vi "fgv_DSP_visa.vi"(7 "action":T1=enum."on", 8 "error in":errorcluster) -> (0 "error out":errorcluster)   [LabVIEW 2019]
uses:
  _ctrl/DSP_action.ctl
  _ctrl/rw.ctl
  _ctrl/init-r-stop.ctl
  SubVIs/common/cmd_err.ctl
  SubVIs/common/Glob_Ref.vi
panel:
  out "Waveform Chart":dbl(graph)
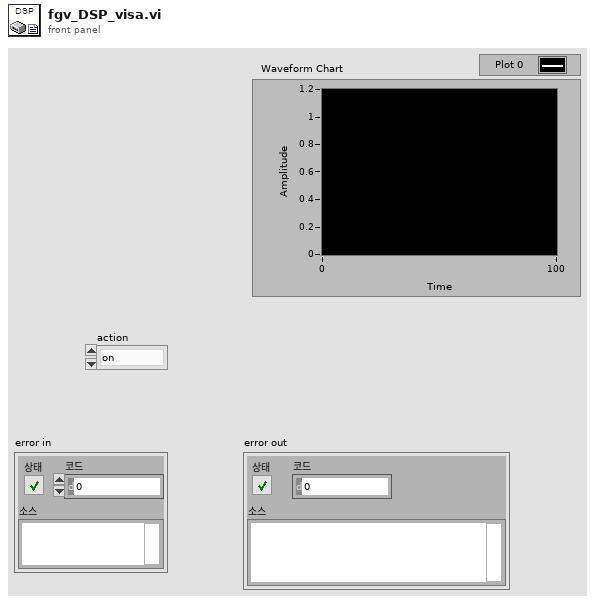
[diagram p1: front panel]
types:
  T1 = typedef "DSP_action.ctl" = enum16{"False", "cont", "on", "off", "discont", "protection", "protection_seq", "preread", "level_seq", "level_m", "read", "stop", "exit"}
  T2 = typedef "rw.ctl" = enum16{"read", "write"}
  T3 = enum16{"DL950", "BP4610", "DSP1500", "cDAQ-AI", "cDAQ-AO", "cDAQ-DO"}
  T4 = typedef "init-r-stop.ctl" = enum16{"ini", "read", "stop"}
  T5 = typedef "cmd_err.ctl" = enum16{"close", "open", "default"}
  T6 = typedef "DSP_config.ctl" = cluster{"Port":refnum<visa-resource-name>, "OVP Level":dbl, "OCP Level":dbl, "Current":dbl, "Voltage":dbl}
  T7 = typedef "DSP_retrun.ctl" = cluster{"voltage":dbl, "current":dbl, "Read Data":string}
  T8 = typedef "cap_config.ctl" = cluster{"Test Mode":enum32{"6.3.2 저온 작동/방치 시험", "6.3.3 고온 작동/방치 시험", "6.3.4 온도 싸이클 시험", "6.3.6 온습도 싸이클 시험", "6.3.8 결로 시험", "6.3.9 빙결 시험", "ON/OFF 동작시험"}, "ON time[ms]":dbl, "OFF time[ms]":dbl, "1. 작동시간[분]":dbl, "2. 미작동시간[분]":dbl, "3. 작동시간[분]":dbl, "level[V]":dbl, "duty":dbl, "Freq":dbl, "Voltage+[V]":dbl, "Voltage-[V]":dbl, "Current+[A]":dbl, "Current-[A]":dbl, "출력전압[V]":dbl, "출력전류[A]":dbl, "OVP Level":dbl, "OCP Level":dbl, "Time Div":u16, "Record Len":i32, "방전 기준[V]":dbl, "Repeate (Each Ch)":u32, "Cycle[N]":u32, "ON/OFF 회 수[N]":dbl, "TrigPos[%]":dbl, "시험시간[분]":dbl}
  T9 = typedef "ref_all.ctl" = cluster{"BP4610 Config":refnum<vi>, "DSP1950 Config":refnum<vi>, "2470-config":refnum<vi>, "cDAQ 9269 AO config":refnum<vi>, "cDAQ 9221 Config":refnum<vi>, "cDAQ-9467 Config":refnum<vi>, "Waveform":refnum<vi>, "DL950 wfm":refnum<vi>, "AI Graph":refnum<vi>, "AO_Wave-config":refnum<vi>, "DL950 items":refnum<vi>, "Volt":refnum<vi>, "Current":refnum<vi>, "AO_Level":refnum<vi>, "RC-Test Judgement ":refnum<vi>, "Log path":refnum<vi>, "시험명":refnum<vi>, "file renew[Hr]":refnum<vi>, "Breakdown-Spec":refnum<vi>, "paste":refnum<vi>, "copy":refnum<vi>, "DL950_config":refnum<vi>, "종료시간":refnum<vi>, "경과시간":refnum<vi>, "Apply":refnum<vi>, "DSP Config LV ":refnum<vi>, "Testconfig":refnum<vi>}
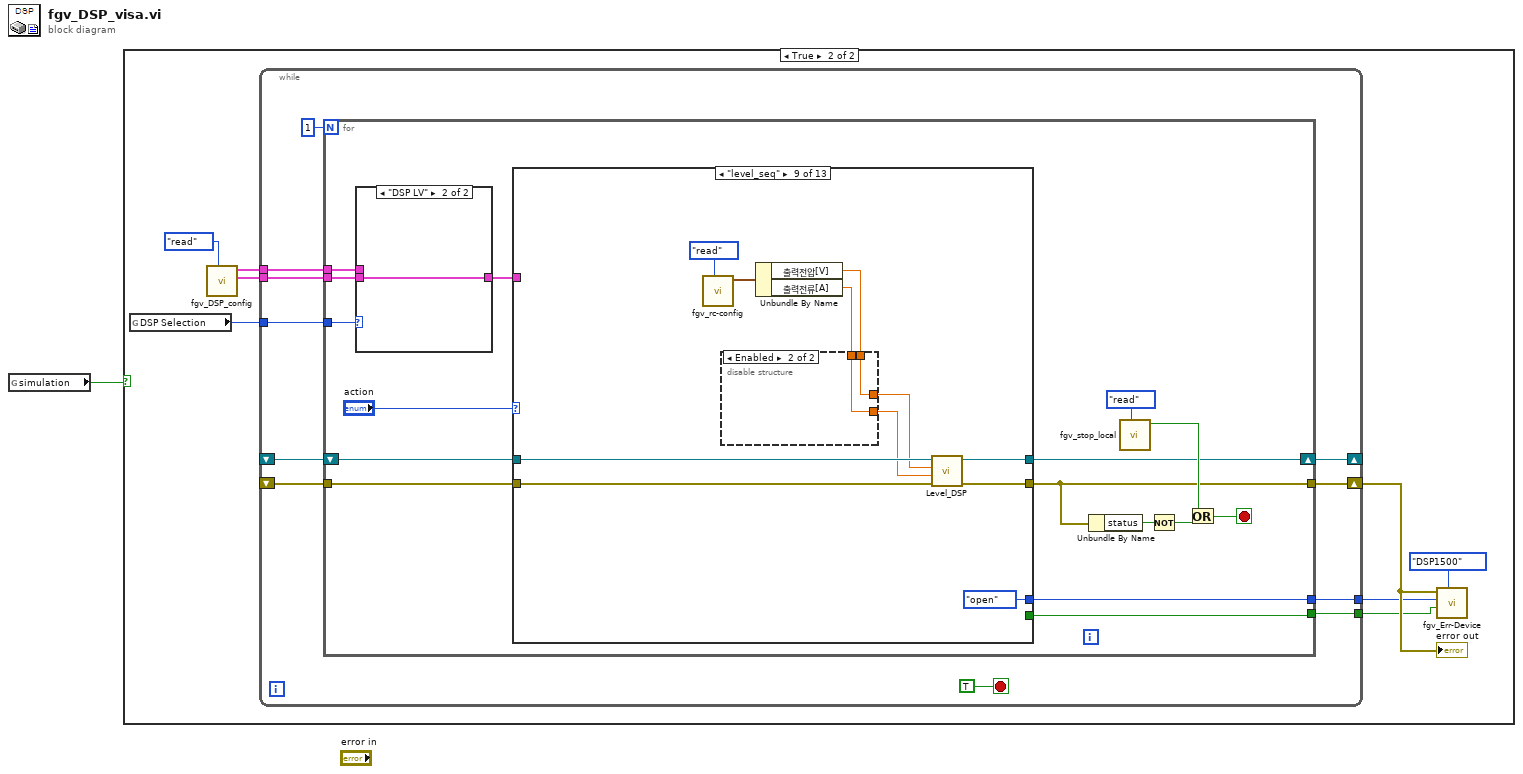
[diagram p0: block diagram]
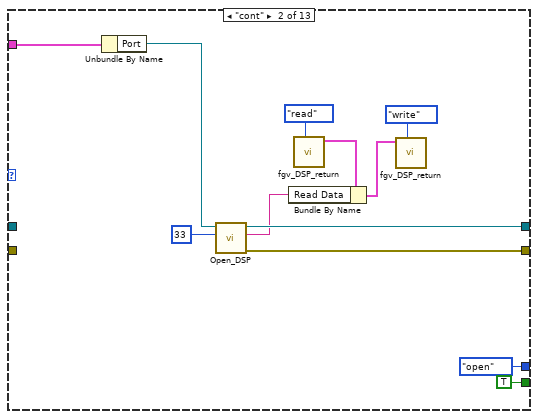
[diagram p5: hidden frame]
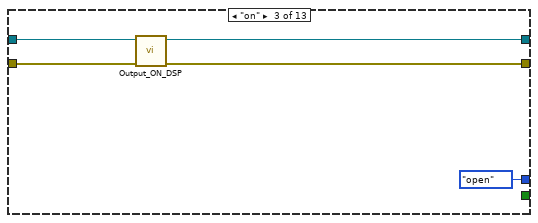
[diagram p6: hidden frame]
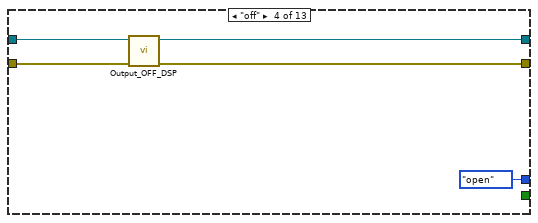
[diagram p7: hidden frame]
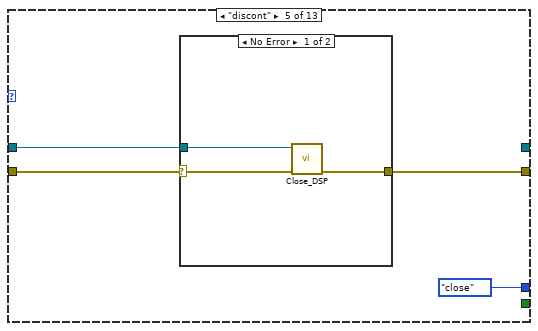
[diagram p8: hidden frame]
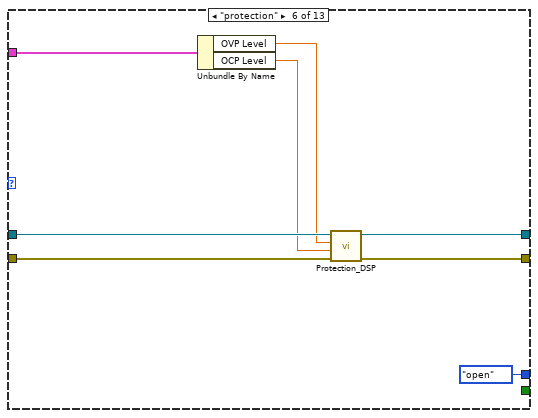
[diagram p10: hidden frame]
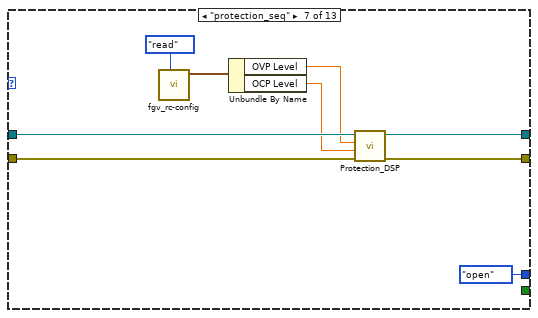
[diagram p11: hidden frame]
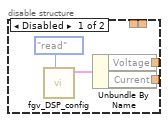
[diagram p13: hidden frame]
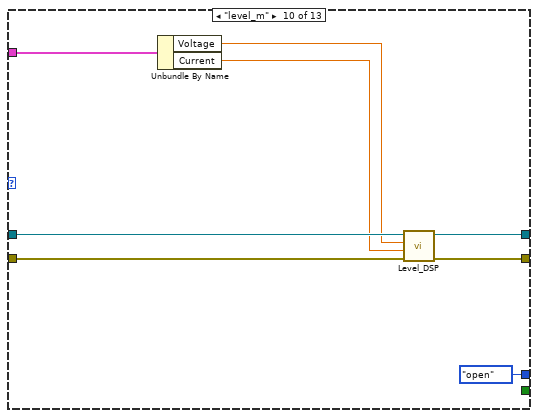
[diagram p14: hidden frame]
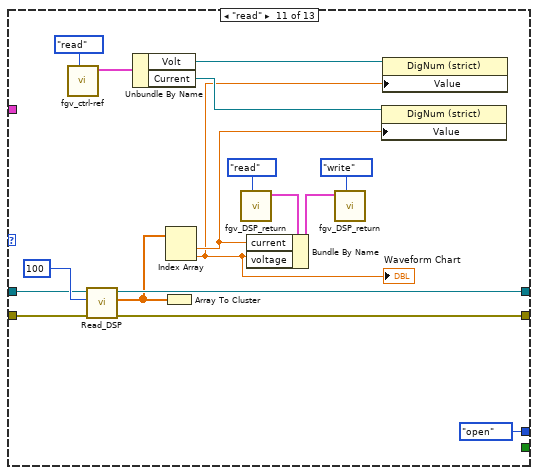
[diagram p15: hidden frame]
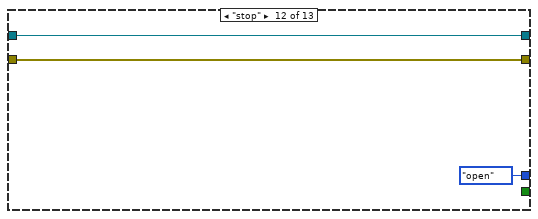
[diagram p16: hidden frame]
diagram:
  n1 = global read "Glob_Ref.vi" "simulation"() -> (w1:bool)
  n2 = case shown="True" w1 {
    frame False {
    }
    frame True {
      n3 = global read "Glob_Ref.vi" "DSP Selection"() -> (w5:enum32{"DSP HV", "DSP LV"})
      n4 = call "fgv_DSP_config.vi"("cmd"=rw."read") -> ("DSP Config LV OUT"=w3:T6, "DSP Config HV OUT"=w2:T6)  [unwired: 8 in, 1 out]
      n5 = while {
        shift-right: [w17] -> _
        shift-left: _ -> [w19]
        shift-right: [w18] -> w8
        shift-left: _ -> [w15]
        tunnel: [w14] -> w7
        tunnel: [w13] -> w6
        tunnel: w5 -> [w12]
        tunnel: w3 -> [w11]
        tunnel: w2 -> [w10]
        stop <- TRUE stop-if-true
        n6 = for {
          N: 1 -> [_]
          tunnel: [w21] -> w18
          shift-right: [w22] -> w17
          shift-left: w19 -> [w35]
          tunnel: w15 -> [w29]
          tunnel: [w28] -> w14
          tunnel: [w27] -> w13
          tunnel: w12 -> [w26]
          tunnel: w11 -> [w25]
          tunnel: w10 -> [w24]
          stop <- w31 stop-if-true
          n7 = case shown="\"DSP LV\"" w26 {
            tunnel: [w37 w38] -> w23
            tunnel: w25 -> [_ w38]
            tunnel: w24 -> [w37 _]
            frame "DSP HV", Default {
            }
            frame "DSP LV" {
            }
          }
          n8 = case shown="\"level_seq\"" "action" {
            tunnel: [w40 w51 w54 w59 w64 w75 w84 w89 w97 w111 w130 w134 w136] -> w21
            tunnel: [w39 w50 w56 w60 _ w76 w85 w88 w98 w112 w129 w133 w135] -> w22
            tunnel: w35 -> [w39 _ w57 w62 w66 w77 w86 w88 w100 w114 w128 w133 w135]
            tunnel: w29 -> [w40 _ w55 w61 w65 w78 w87 w89 w99 w113 w127 w134 w136]
            tunnel: [_ cmd_err."open" ("cmd") cmd_err."open" ("cmd") cmd_err."open" ("cmd") cmd_err."close" ("cmd") cmd_err."open" ("cmd") cmd_err."open" ("cmd") _ cmd_err."open" ("cmd") cmd_err."open" ("cmd") cmd_err."open" ("cmd") cmd_err."open" ("cmd") _] -> w28
            tunnel: [_ TRUE ("first?") _ _ _ _ _ _ _ _ _ _ _] -> w27
            tunnel: w23 -> [_ w41 _ _ _ w71 _ _ _ w107 _ _ _]
            frame "False", Default {
            }
            frame "cont" {
              n9 = Unbundle By Name(w41) -> ("Port"=w49:refnum<visa-resource-name>)
              n10 = call "Open_DSP.vi"("Byte count"=u32 33, "VISA"=w49) -> ("error out"=w51:errorcluster, "read buffer"=w45:string, "VISA out"=w50:refnum<visa-resource-name>)  [unwired: 7 in]
              n11 = call "fgv_DSP_return.vi"("cmd"=rw."read") -> ("return 2"=w46:T7)  [unwired: 9 in, 1 out]
              n12 = Bundle By Name(cluster=w46, "Read Data"=w45) -> (w44:T7)
              n13 = call "fgv_DSP_return.vi"("cmd"=rw."write", "return"=w44) -> ()  [unwired: 8 in, 2 out]
            }
            frame "on" {
              n14 = call "Output_ON_DSP.vi"("error in"=w55, "VISA"=w57) -> ("error out"=w54:errorcluster, "VISA  Out"=w56:refnum<visa-resource-name>)  [unwired: 8 in]
            }
            frame "off" {
              n15 = call "Output_OFF_DSP.vi"("error in"=w61, "VISA"=w62) -> ("error out"=w59:errorcluster, "VISA2"=w60:refnum<visa-resource-name>)  [unwired: 8 in]
            }
            frame "discont" {
              n16 = case shown="No Error" w65 {
                selector: w65 -> [w68 w70]
                tunnel: w66 -> [w69 _]
                tunnel: [w67 w70] -> w64
                frame No Error {
                  n17 = call "Close_DSP.vi"("error in (no error)"=w68, "VISA resource name"=w69) -> ("error out"=w67:errorcluster)  [unwired: 9 in]
                }
                frame Error {
                }
              }
            }
            frame "protection" {
              n18 = Unbundle By Name(w71) -> ("OVP Level"=w73:dbl, "OCP Level"=w74:dbl)
              n19 = call "Protection_DSP.vi"("error in (no error)"=w78, "OCP Level"=w74, "OVP Level"=w73, "VISA resource name"=w77) -> ("error out"=w75:errorcluster, "VISA resource name Out"=w76:refnum<visa-resource-name>)  [unwired: 6 in]
            }
            frame "protection_seq" {
              n20 = call "fgv_rc-config.vi"("cmd"=rw."read") -> ("Testconfig out"=w80:T8)  [unwired: 9 in, 1 out]
              n21 = Unbundle By Name(w80) -> ("OVP Level"=w82:dbl, "OCP Level"=w83:dbl)
              n22 = call "Protection_DSP.vi"("error in (no error)"=w87, "OCP Level"=w83, "OVP Level"=w82, "VISA resource name"=w86) -> ("error out"=w84:errorcluster, "VISA resource name Out"=w85:refnum<visa-resource-name>)  [unwired: 6 in]
            }
            frame "preread" {
            }
            frame "level_seq" {
              n23 = call "fgv_rc-config.vi"("cmd"=rw."read") -> ("Testconfig out"=w93:T8)  [unwired: 9 in, 1 out]
              n24 = Unbundle By Name(w93) -> ("출력전압[V]"=w92:dbl, "출력전류[A]"=w91:dbl)
              n25 = disable-structure shown="Enabled" {
                disable-tunnel: [w102 w106] -> w96
                disable-tunnel: [w101 w105] -> w95
                disable-tunnel: w92 -> [_ w106]
                disable-tunnel: w91 -> [_ w105]
                frame Disabled {
                  n26 = call "fgv_DSP_config.vi"("cmd"=rw."read") -> ("DSP Config HV OUT"=w103:T6)  [unwired: 8 in, 2 out]
                  n27 = Unbundle By Name(w103) -> ("Voltage"=w102:dbl, "Current"=w101:dbl)
                }
                frame Enabled {
                }
              }
              n28 = call "Level_DSP.vi"("error in (no error)"=w99, "Curr"=w95, "Volt"=w96, "VISA resource name"=w100) -> ("error out"=w97:errorcluster, "VISA resource name Out"=w98:refnum<visa-resource-name>)  [unwired: 6 in]
            }
            frame "level_m" {
              n29 = Unbundle By Name(w107) -> ("Voltage"=w110:dbl, "Current"=w109:dbl)
              n30 = call "Level_DSP.vi"("error in (no error)"=w113, "Curr"=w109, "Volt"=w110, "VISA resource name"=w114) -> ("error out"=w111:errorcluster, "VISA resource name Out"=w112:refnum<visa-resource-name>)  [unwired: 6 in]
            }
            frame "read" {
              n31 = call "fgv_ctrl-ref.vi"("cmd"=rw."read") -> ("output cluster 2"=w120:T9)  [unwired: 9 in, 1 out]
              n32 = call "Read_DSP.vi"("error in"=w127, "Byte count"=u32 100, "port"=w128) -> ("error out"=w130:errorcluster, "Data"=w122:dbl[], "port Out"=w129:refnum<visa-resource-name>)  [unwired: 6 in]
              n33 = Unbundle By Name(w120) -> ("Volt"=w119:refnum<vi>, "Current"=w118:refnum<vi>)
              n34 = Array To Cluster(array=w122) -> ()  [unwired: 1 out]
              n35 = Index Array(array=w122) -> (element #1=w117:dbl, element #2=w116:dbl)  [unwired: 2 in]
              "Waveform Chart" <- w116
              n36 = call "fgv_DSP_return.vi"("cmd"=rw."read") -> ("return 2"=w124:T7)  [unwired: 9 in, 1 out]
              n37 = Bundle By Name(cluster=w124, "current"=w117, "voltage"=w116) -> (w123:T7)
              n38 = call "fgv_DSP_return.vi"("cmd"=rw."write", "return"=w123) -> ()  [unwired: 8 in, 2 out]
              n39 = property class="DigNum (strict)"(reference=w118, "Value"=w117) -> ()  [unwired: 1 in, 2 out]
              n40 = property class="DigNum (strict)"(reference=w119, "Value"=w116) -> ()  [unwired: 1 in, 2 out]
            }
            frame "stop" {
            }
            frame "exit" {
            }
          }
          n41 = Unbundle By Name(w21) -> ("status"=w33:bool)
          n42 = call "fgv_stop_local.vi"("cmd"=init-r-stop."read") -> ("stop"=w30:bool)  [unwired: 9 in, 1 out]
          n43 = Not(x=w33) -> (.not. x?=w32:bool)
          n44 = Or(x=w30, y=w32) -> (x .or. y?=w31:bool)
        }
      }
      "error out" <- w8
      n45 = call "fgv_Err-Device.vi"("Err Sel"=T3."DSP1500", "first?"=w6, "cmd"=w7, "error in"=w8) -> ()  [unwired: 8 in]
    }
  }
